vi "FPGA Main V3.vi"() -> ()   [LabVIEW 2018]
doc: "This VI reads all analogue data channels available at the fastest rate supported by the respective hardware and updates a memory address for when each measurement is available.\n\nAt a rate defined by the fastest module (NI 9237 - default of 12.5kHz) this memory is read, combined with the measurements from the 9237 module and written to the FIFO for communication to the RT machine.\n\nThe NI 9237 modeul therefore defines the nominal sampling rate of the system (with slower channels over-sampled).\n\nA time channel (in uSec) is provided with 0 referenced from the first acquisition of the NI 9237 module"
uses:
  <vilib>/LabVIEW Targets/FPGA/cRIO/shared/nicrio_ModuleControls/nicrio_cRIO-9237_DataRatesRing.ctl
  <vilib>/Platform/TimedLoop/XDataNode/timing_clust.ctl
  <vilib>/Platform/TimedLoop/XDataNode/nitl_modes.ctl
  <vilib>/Platform/TimedLoop/XDataNode/wakeup.ctl
  <vilib>/rvi/Emulation/niFpgaGetClockAttributes.vi
  <vilib>/rvi/Emulation/niFpgaSctlEmulationGetInTimedLoop.vi
  <vilib>/rvi/Emulation/niFpgaEmulationReportErrorSimple.vi
  <vilib>/rvi/Emulation/niFpgaProcessEmulError.vi
  <vilib>/rvi/eio/common/nirviEmuTemplatePropertySet_noerrors.vi
  <vilib>/rvi/eio/common/nirviEmuTemplateMethod_errors.vi
  <vilib>/rvi/interface/RandomDataEmulation/niFpgaRandomDataHandleErrors.vi
  <vilib>/rvi/Memory/Memory_Emulation/nirvimemoryFastEmulation.vi
  <vilib>/rvi/Memory/Memory_Emulation/nirvimemoryEmulation.vi
  <vilib>/rvi/Emulation/niFpgaEmulationIsFPGAContextNoSignature.vi
  <vilib>/rvi/DataTransferAndStorage/Container/Common/niFpgaContainerGetUniqueNameForEmu.vi
  <vilib>/rvi/errors/nirviReportUnexpectedCaseInternalError (U32).vi
  <vilib>/rvi/Emulation/niFpgaCriticalErrorInLSC.vi
  <vilib>/rvi/FIFO/Fifo_Resource/nirvififoEmulationSetSize.vi
  <vilib>/rvi/FIFO/Fifo_Resource/nirviFifoEmulationQueueMgr.vi
  <instcachedir>/0/nirviFifoEmulationQueueMgr_E5CAEC123FF24DC58D834DCA3CDAA9B5.lvgen/nirviFifoEmulationQueueMgr_E5CAEC123FF24DC58D834DCA3CDAA9B5_002.vi
  <vilib>/rvi/errors/niFpgaSetErrorForExecOnDevCompSimple.vi
  <vilib>/rvi/eio/common/nirviEmuReportErrorAndStop.vi
  <vilib>/Utility/error.llb/Clear Errors.vi
  <vilib>/rvi/FIFO/Fifo_Resource/nirvififoEmulationCreateLock.vi
  <vilib>/rvi/FIFO/Fifo_Resource/nirvififoEmulationObtainLock.vi
  <vilib>/rvi/FIFO/Fifo_Resource/nirvififoEmulationReleaseLock.vi
  <vilib>/rvi/occurrence/nirviWaitOnOccurrenceBase.vi
  <vilib>/rvi/errors/nirviReportUnexpectedCaseInternalError.vi
  <vilib>/rvi/FIFO/Fifo_Resource/nirvififoEmulationDetermineInputValidOut.vi
  <vilib>/eio/EIOPropertyNode/EIOPropertyNode.xnode
  <vilib>/eio/EIONode/EIONode.xnode
  <vilib>/rvi/DataTransferAndStorage/Container/XNode/niFpgaContainer.xnode
  <vilib>/rvi/interface/RandomDataEmulation/nirviRandomDataFpgaReadWriteTemplate.vi
  <vilib>/rvi/FIFO/Fifo_Resource/nirvififoEmulationGetNumberOfElementsToRead.vi
  <vilib>/rvi/FIFO/Fifo_Resource/nirvififoEmulationRead.vi
  <vilib>/eio/EIOMethodNode/EIOMethodNode.xnode
  <vilib>/platform/TimedLoop/XDataNode/XDataNode.xnode
  <vilib>/rvi/FIFO/Fifo_Resource/nirvififoEmulationWrite.vi
  <vilib>/Platform/TimedLoop/XDataNode/XDNodeRunTimeDep.lvlib
  <vilib>/rvi/eio/common/nirviEmuTemplatePropertyGet_errors.vi
  <vilib>/rvi/eio/common/nirviEmuTemplatePropertyGet_noerrors.vi
  <vilib>/rvi/eio/common/nirviEmuTemplatePropertySet_errors.vi
panel:
  in  "speedOutputScaling":sgl=6366198.0
  out "Speed":sgl caption="Speed (rads/tick)"
  out "filteredAngle":sgl caption="filteredAngle (rads)"
  out "filteredSpeed":sgl
  out "S1":u32
  in  "Edge filter":T1={"filterSize"=50, "lowerThreshold"=5, "upperThreshold"=45}
  out "edge separation":u32 caption="edge separation (ticks)"
  in  "falling edge (F)":bool caption="Torque encoder direction"
  in  "switch encoders":bool
  in  "Data Rate":T2=1 items=["50.000 kS/s (NI 9237)"=1, "25.000 kS/s (NI 9237)"=2, "16.667 kS/s (NI 9237)"=3, "12.500 kS/s (NI 9237)"=4, "10.000 kS/s (NI 9237)"=5, "8.333 kS/s (NI 9237)"=6, "7.143 kS/s (NI 9237)"=7, "6.250 kS/s (NI 9237)"=8, "5.556 kS/s (NI 9237)"=9, "5.000 kS/s (NI 9237)"=10, "4.545 kS/s (NI 9237)"=11, "4.167 kS/s (NI 9237)"=12, "3.846 kS/s (NI 9237)"=13, "3.571 kS/s (NI 9237)"=14, "3.333 kS/s (NI 9237)"=15, "3.125 kS/s (NI 9237)"=16, "2.941 kS/s (NI 9237)"=17, "2.778 kS/s (NI 9237)"=18, "2.632 kS/s (NI 9237)"=19, "2.500 kS/s (NI 9237)"=20, "2.381 kS/s (NI 9237)"=21, "2.273 kS/s (NI 9237)"=22, "2.174 kS/s (NI 9237)"=23, "2.083 kS/s (NI 9237)"=24, "2.000 kS/s (NI 9237)"=25, "1.923 kS/s (NI 9237)"=26, "1.852 kS/s (NI 9237)"=27, "1.786 kS/s (NI 9237)"=28, "1.724 kS/s (NI 9237)"=29, "1.667 kS/s (NI 9237)"=30, "1.613 kS/s (NI 9237)"=31]
  out "Total channel count":u32=61
  out "timestamp":u32
  out "FIFO full counter":i32
  in  "Safe Voltage":fxp<+/-,20,5>[](array[numeric])=[0.0, 0.0, 0.0, 0.0]
  in  "Safe Digital":bool[](array[boolean])=[FALSE, FALSE, FALSE, FALSE, FALSE, FALSE, FALSE, FALSE]
  in  "Voltage Out":fxp<+/-,20,5>[](array[numeric])=[0.0, 0.0, 0.0, 0.0]
  in  "Update Outputs":bool
  in  "Mod 8":bool[](array[boolean])=[FALSE, FALSE, FALSE, FALSE, FALSE, FALSE, FALSE, FALSE]
  out "E Stop":bool
  in  "Stop acquire":bool
  # "Torque Measurement"
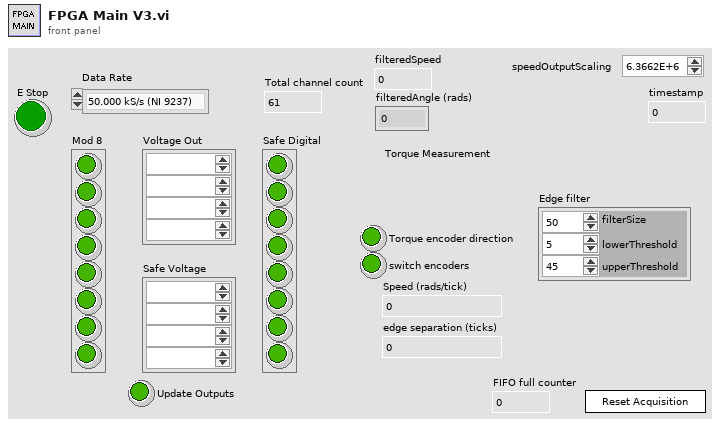
[diagram p1: front panel]
types:
  T1 = cluster{"filterSize":u8, "lowerThreshold":u8, "upperThreshold":u8}
  T2 = typedef "nicrio_cRIO-9237_DataRatesRing.ctl" = u8
  T3 = typedef "XDNodeRunTimeDep.lvlib/timing_clust.ctl" = cluster{"Expected End [f-1]":u64, "Actual End [f-1]":u64, "Finished Late? [f-1]":bool, "Expected End [i-1]":u64, "Actual End [i-1]":u64, "Finished Late? [i-1]":bool, "Expected Start [i]":u64, "Actual Start [i]":u64, "Expected Start [f]":u64, "Actual Start [f]":u64, "Source Name":string, "Structure Name":string, "Period":i64, "Deadline":i64, "Offset":i64, "Start":i64, "Priority":i32, "Timeout":i32, "Mode":T4, "Wakeup Reason":T5, "Error":errorcluster, "Source Type":string, "Secondary Source Type":string, "Global End Time":u64, "Global Start Time":u64, "Frame Duration":u64, "Iteration Duration":u64, "Assigned CPU":i32, "I/O Scan Engine Mode":u32}
  T4 = typedef "XDNodeRunTimeDep.lvlib/nitl_modes.ctl" = enum32{"No Change", "Process missed periods, maintain original phase", "Discard missed periods, maintain original phase", "Process missed periods, ignore original phase", "Discard missed periods, ignore original phase"}
  T5 = typedef "XDNodeRunTimeDep.lvlib/wakeup.ctl" = enum32{"Normal", "Aborted", "Asynchronous wakeup", "Timing source error", "Timed loop error", "Timeout"}
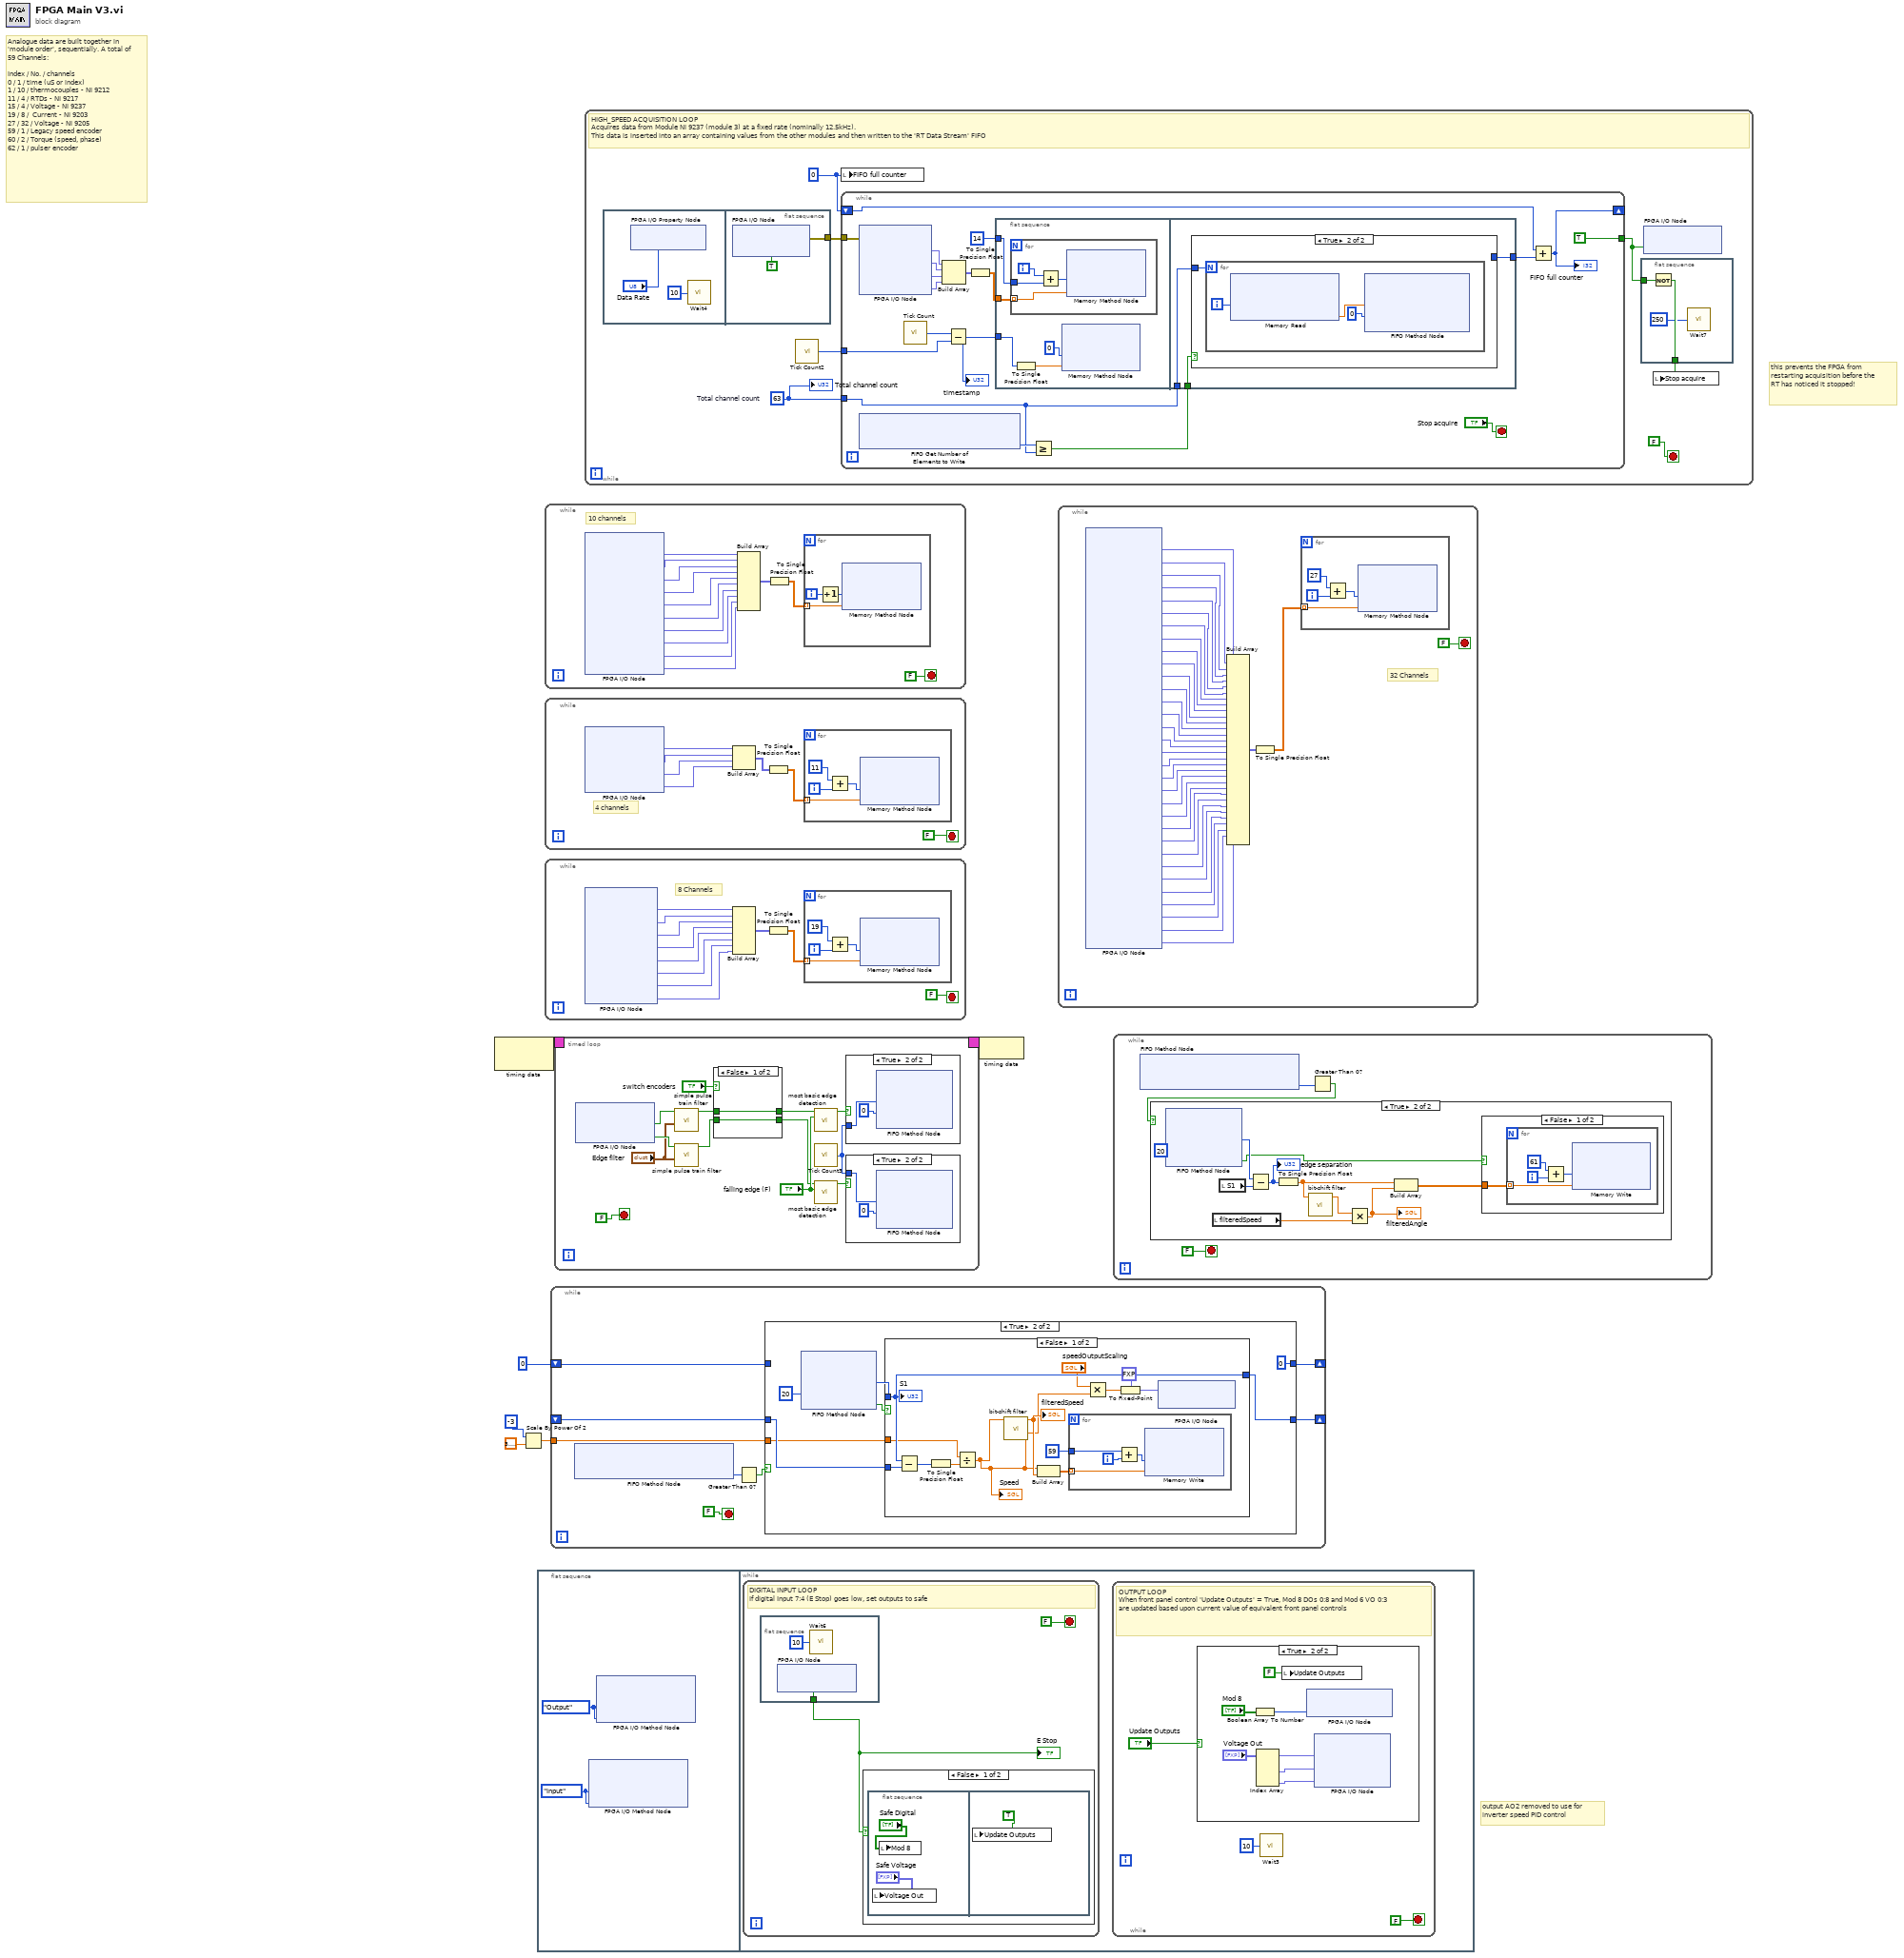
[diagram p0: block diagram]
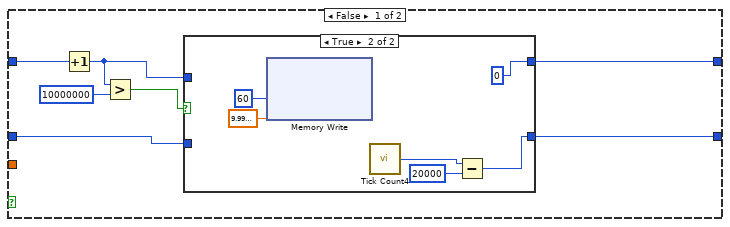
[diagram p4: hidden frame]
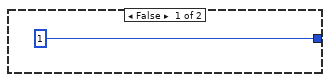
[diagram p12: hidden frame]
diagram:
  # "output AO2 removed to use for inverter speed PID control"
  # "this prevents the FPGA from restarting acquisition before the RT has noticed it stopped!"
  # "Analogue data are built together in 'module order', sequentially. A total of 59 Channels:\n\nIndex / No. / channels\n0 / 1 / time (uS or index)\n1 / 10 / thermocouples - NI 9212\n11 / 4 / RTDs - NI 9217\n15 / 4 / Voltage - NI 9237\n19 / 8 /  Current - NI 9203\n27 / 32 / Voltage - NI 9205\n59 / 1 / Legacy speed encoder\n60 / 2 / Torque (speed, phase)\n62 / 1 / pulser encoder"
  n1 = node-c288() -> (w6:T3)  [unwired: 1 in]
  n2 = Scale By Power Of 2(n=i16 -3, x=sgl 3.1415927) -> (x*2^n=w2:sgl)
  n3 = flat-sequence {
    frame #0 {
      w7 = enum8{"No Change", "Input", "Output"}."Output" ("DIO 7:4")
      w8 = enum8{"No Change", "Input", "Output"}."Input" ("DIO 7:4")
      n4 = xnode "FPGA I/O Method Node"("DIO 7:4"=w8, "DIO 3:0"=w8) -> ()  [unwired: 1 in, 1 out]
      n5 = xnode "FPGA I/O Method Node"("DIO 7:4"=w7, "DIO 3:0"=w7) -> ()  [unwired: 1 in, 1 out]
    }
    frame #1 {
      n6 = while {
        stop <- FALSE stop-if-true
        # "DIGITAL INPUT LOOP\nIf digital Input 7:4 (E Stop) goes low, set outputs to safe"
        n7 = flat-sequence {
          tunnel: [w22] -> w19
          frame #0 {
            n8 = xnode "FPGA I/O Node"() -> ("Mod7/DIO4"=w22:bool)  [unwired: 1 in, 1 out]
            n9 = call "Wait6"("Count(uSec)"=u8 10) -> ()  [unwired: 1 out]
          }
        }
        n10 = case shown="False" w19 {
          frame False {
            n11 = flat-sequence {
              frame #0 {
                n12 = local write "Voltage Out"("Safe Voltage") -> ()
                n13 = local write "Mod 8"("Safe Digital") -> ()
              }
              frame #1 {
                n14 = local write "Update Outputs"(TRUE ("Update Outputs")) -> ()
              }
            }
          }
          frame True {
          }
        }
        "E Stop" <- w19
      }
      n15 = while {
        stop <- FALSE stop-if-true
        # "OUTPUT LOOP\nWhen front panel control 'Update Outputs' = True, Mod 8 DOs 0:8 and Mod 6 VO 0:3 are updated based upon current value of equivalent front panel controls"
        n16 = case shown="True" "Update Outputs" {
          frame False {
          }
          frame True {
            n17 = Boolean Array To Number(Boolean array="Mod 8") -> (number=w17:u8)
            n18 = Index Array(array="Voltage Out") -> (element #1=w15:fxp<+/-,20,5>, element #2=w14:fxp<+/-,20,5>, element #4=w13:fxp<+/-,20,5>)  [unwired: 4 in, 1 out]
            n19 = local write "Update Outputs"(FALSE ("Update Outputs")) -> ()
            n20 = xnode "FPGA I/O Node"("Mod8/DIO7:0"=w17) -> ()  [unwired: 1 in, 1 out]
            n21 = xnode "FPGA I/O Node"("Mod6/AO0"=w15, "Mod6/AO1"=w14, "Mod6/AO3"=w13) -> ()  [unwired: 3 in, 3 out]
          }
        }
        n22 = call "Wait3"("Count(uSec)"=u16 10 ("Count(Ticks)")) -> ()  [unwired: 1 out]
      }
    }
  }
  n23 = while {
    stop <- FALSE stop-if-true
    # "10 channels"
    n24 = xnode "FPGA I/O Node"() -> ("Mod1/TC0"=w38:fxp<+/-,24,-2>, "Mod1/TC1"=w37:fxp<+/-,24,-2>, "Mod1/TC2"=w36:fxp<+/-,24,-2>, "Mod1/TC3"=w35:fxp<+/-,24,-2>, "Mod1/TC4"=w34:fxp<+/-,24,-2>, "Mod1/TC5"=w33:fxp<+/-,24,-2>, "Mod1/TC6"=w32:fxp<+/-,24,-2>, "Mod1/TC7"=w31:fxp<+/-,24,-2>, "Mod1/CJC0"=w28:fxp<+/-,24,-2>, "Mod1/CJC1"=w27:fxp<+/-,24,-2>)  [unwired: 10 in, 10 out]
    n25 = Build Array(w38, w37, w36, w35, w34, w33, w32, w31, w28, w27) -> (w30:fxp<+/-,24,-2>[])
    n26 = To Single Precision Float(number=w30) -> (single precision float=w29:sgl[])
    n27 = for {
      tunnel: w29 -> [w41] mode=indexing
      i -> [w40]
      n28 = Increment(x=w40) -> (x+1=w39:i32)
      n29 = xnode ("Memory Method Node")("Address"=w39, "Data"=w41) -> ()  [unwired: 1 in, 1 out]
    }
  }
  n30 = while {
    stop <- FALSE stop-if-true
    # "4 channels"
    n31 = xnode "FPGA I/O Node"() -> ("Mod2/RTD0"=w48:fxp<+/-,24,10>, "Mod2/RTD1"=w47:fxp<+/-,24,10>, "Mod2/RTD2"=w46:fxp<+/-,24,10>, "Mod2/RTD3"=w43:fxp<+/-,24,10>)  [unwired: 4 in, 4 out]
    n32 = Build Array(w48, w47, w46, w43) -> (w45:fxp<+/-,24,10>[])
    n33 = To Single Precision Float(number=w45) -> (single precision float=w44:sgl[])
    n34 = for {
      tunnel: w44 -> [w52] mode=indexing
      i -> [w51]
      n35 = Add(x=11 ("Numeric"), y=w51) -> (x+y=w50:i32)
      n36 = xnode ("Memory Method Node")("Address"=w50, "Data"=w52) -> ()  [unwired: 1 in, 1 out]
    }
  }
  n37 = while {
    stop <- FALSE stop-if-true
    # "8 Channels"
    n38 = xnode "FPGA I/O Node"() -> ("Mod4/AI0"=w63:fxp<+/-,21,-4>, "Mod4/AI1"=w62:fxp<+/-,21,-4>, "Mod4/AI2"=w61:fxp<+/-,21,-4>, "Mod4/AI3"=w58:fxp<+/-,21,-4>, "Mod4/AI4"=w57:fxp<+/-,21,-4>, "Mod4/AI5"=w56:fxp<+/-,21,-4>, "Mod4/AI6"=w55:fxp<+/-,21,-4>, "Mod4/AI7"=w54:fxp<+/-,21,-4>)  [unwired: 8 in, 8 out]
    n39 = Build Array(w63, w62, w61, w58, w57, w56, w55, w54) -> (w60:fxp<+/-,21,-4>[])
    n40 = To Single Precision Float(number=w60) -> (single precision float=w59:sgl[])
    n41 = for {
      tunnel: w59 -> [w67] mode=indexing
      i -> [w66]
      n42 = Add(x=19 ("Numeric"), y=w66) -> (x+y=w65:i32)
      n43 = xnode ("Memory Method Node")("Address"=w65, "Data"=w67) -> ()  [unwired: 1 in, 1 out]
    }
  }
  n44 = while {
    shift-right: [w74] -> _
    shift-left: _ -> [w73]
    tunnel: w2 -> [w72]
    shift-right: [w68] -> _
    shift-left: u32 0 ("n") -> [w69]
    stop <- FALSE stop-if-true
    n45 = xnode ("FIFO Method Node")() -> ("Number of Elements to Read"=w71:u32)  [unwired: 1 in, 1 out]
    n46 = Greater Than 0?(x=w71) -> (x > 0?=w70:bool)
    n47 = case shown="True" w70 {
      tunnel: [w76 w92] -> w74
      tunnel: w73 -> [w80 w97]
      tunnel: w72 -> [_ w96]
      tunnel: w69 -> [w82 _]
      tunnel: [w77 u32 0 ("n")] -> w68
      frame False {
        n48 = Increment(x=w82) -> (x+1=w78:u32)
        n49 = Greater?(x=w78, y=u32 10000000) -> (0:w79:bool)
        n50 = case shown="True" w79 {
          tunnel: w80 -> [w83 _]
          tunnel: w78 -> [w84 _]
          tunnel: [w84 u32 0 ("n")] -> w77
          tunnel: [w83 w86] -> w76
          frame False {
          }
          frame True {
            n51 = xnode ("Memory Write")("Address"=u32 60, "Data"=sgl 1e-09) -> ()  [unwired: 1 in, 1 out]
            n52 = call "Tick Count4"() -> ("Tick Count(Ticks)"=w89:u32)
            n53 = Subtract(x=w89, y=u32 20000) -> (x-y=w86:u32)
          }
        }
      }
      frame True {
        n54 = xnode ("FIFO Method Node")("Timeout"=20) -> ("Element"=w94:u32, "Timed Out?"=w93:bool)  [unwired: 1 in, 1 out]
        n55 = case shown="False" w93 {
          tunnel: w97 -> [w110 w115]
          tunnel: w96 -> [w107 _]
          tunnel: w94 -> [w108 _]
          tunnel: [w108 w115] -> w92
          frame False {
            n56 = Subtract(x=w108, y=w110) -> (x-y=w106:u32)
            n57 = To Single Precision Float(number=w106) -> (single precision float=w105:sgl)
            n58 = Divide(x=w107, y=w105) -> (x/y=w98:sgl)
            "Speed" <- w98
            n59 = call "bit-shift filter.vi"("newValue"=w98) -> ("filteredValue"=w103:sgl)  [unwired: 10 in]
            "filteredSpeed" <- w103
            n60 = Build Array(w98, w103) -> (w104:sgl[])
            n61 = for {
              tunnel: u32 59 ("Address") -> [w114]
              tunnel: w104 -> [w113] mode=indexing
              i -> [w111]
              n62 = Add(x=w114, y=w111) -> (x+y=w112:u32)
              n63 = xnode ("Memory Write")("Address"=w112, "Data"=w113) -> ()  [unwired: 1 in, 1 out]
            }
            n64 = Multiply(x="speedOutputScaling", y=w98) -> (x*y=w101:sgl)
            n65 = To Fixed-Point(fixed-point type=fxp<+/-,20,5> 0.0 ("Mod6/AO2"), number=w101) -> (fixed-point=w100:fxp<+/-,20,5>)
            n66 = xnode "FPGA I/O Node"("Mod6/AO2"=w100) -> ()  [unwired: 1 in, 1 out]
            "S1" <- w108
          }
          frame True {
          }
        }
      }
    }
  }
  n67 = timed-loop {
    timing: w6 -> [_]
    timing-out: [_] -> w5
    stop <- FALSE stop-if-true
    n68 = xnode "FPGA I/O Node"() -> ("Mod7/DIO0"=w128:bool, "Mod7/DIO1"=w127:bool)  [unwired: 2 in, 2 out]
    n69 = call "simple pulse train filter.vi"("filter params"="Edge filter", "realState"=w128) -> ("filteredState"=w120:bool)  [unwired: 9 in]
    n70 = call "simple pulse train filter.vi"("filter params"="Edge filter", "realState"=w127) -> ("filteredState"=w122:bool)  [unwired: 9 in]
    n71 = case shown="False" "switch encoders" {
      tunnel: [w134 w135] -> w123
      tunnel: w122 -> [w134 w136]
      tunnel: [w133 w136] -> w121
      tunnel: w120 -> [w133 w135]
      frame False {
      }
      frame True {
      }
    }
    n72 = call "most basic edge detection.vi"("falling edge"="falling edge (F)", "pulse"=w121) -> ("edge detected"=w119:bool)  [unwired: 9 in]
    n73 = call "Tick Count3"() -> ("Tick Count(Ticks)"=w116:u32)
    n74 = call "most basic edge detection.vi"("falling edge"="falling edge (F)", "pulse"=w123) -> ("edge detected"=w117:bool)  [unwired: 9 in]
    n75 = case shown="True" w119 {
      tunnel: w116 -> [_ w132]
      frame False {
      }
      frame True {
        n76 = xnode ("FIFO Method Node")("Element"=w132, "Timeout"=0) -> ()  [unwired: 1 in, 2 out]
      }
    }
    n77 = case shown="True" w117 {
      tunnel: w116 -> [_ w130]
      frame False {
      }
      frame True {
        n78 = xnode ("FIFO Method Node")("Element"=w130, "Timeout"=0) -> ()  [unwired: 1 in, 2 out]
      }
    }
  }
  n79 = while {
    stop <- FALSE stop-if-true
    w140 = 0 ("FIFO full counter")
    w143 = u32 63  # Total channel count
    # "HIGH_SPEED ACQUISITION LOOP\nAcquires data from Module NI 9237 (module 3) at a fixed rate (nominally 12.5kHz).\nThis data is inserted into an array containing values from the other modules and then written to the 'RT Data Stream' FIFO"
    n80 = flat-sequence {
      tunnel: [w152] -> w144
      frame #0 {
        n81 = xnode "FPGA I/O Property Node"("Data Rate"="Data Rate") -> ()  [unwired: 1 in, 1 out]
        n82 = call "Wait4"("Count(mSec)"=u16 10) -> ()  [unwired: 1 out]
      }
      frame #1 {
        n83 = xnode "FPGA I/O Node"("Mod3/Start"=TRUE) -> ("error out"=w152:errorcluster)  [unwired: 2 in, 1 out]
      }
    }
    n84 = call "Tick Count2"() -> ("Tick Count(uSec)"=w145:u32)
    n85 = local write "FIFO full counter"(w140) -> ()
    n86 = while {
      tunnel: [TRUE ("I/O Item")] -> w142
      tunnel: w144 -> [w170]
      tunnel: w143 -> [w155]
      shift-right: [w163] -> _
      shift-left: w140 -> [w161]
      tunnel: w145 -> [w164]
      stop <- "Stop acquire" stop-if-true
      n87 = xnode "FPGA I/O Node"("error in"=w170) -> ("Mod3/AI0"=w169:fxp<+/-,24,-4>, "Mod3/AI1"=w168:fxp<+/-,24,-4>, "Mod3/AI2"=w167:fxp<+/-,24,-4>, "Mod3/AI3"=w166:fxp<+/-,24,-4>)  [unwired: 4 in, 5 out]
      n88 = xnode ("FIFO Get Number of Elements to Write")() -> ("Number of Elements to Write"=w157:u32)  [unwired: 1 in, 1 out]
      n89 = call "Tick Count"() -> ("Tick Count(uSec)"=w160:u32)
      n90 = Build Array(w169, w168, w167, w166) -> (w165:fxp<+/-,24,-4>[])
      n91 = Subtract(x=w160, y=w164) -> (x-y=w153:u32)
      "timestamp" <- w153
      n92 = To Single Precision Float(number=w165) -> (single precision float=w159:sgl[])
      n93 = flat-sequence {
        tunnel: w159 -> [w176]
        tunnel: 14 ("index") -> [w175]
        tunnel: w153 -> [w173]
        tunnel: w155 -> [w183]
        tunnel: [w182] -> w154
        tunnel: w156 -> [w181]
        frame #0 {
          n94 = for {
            tunnel: w176 -> [w180] mode=indexing
            tunnel: w175 -> [w179]
            i -> [w177]
            n95 = Add(x=w177, y=w179) -> (x+y=w178:i32)
            n96 = xnode ("Memory Method Node")("Address"=w178, "Data"=w180) -> ()  [unwired: 1 in, 1 out]
          }
          n97 = To Single Precision Float(number=w173) -> (single precision float=w174:sgl)
          n98 = xnode ("Memory Method Node")("Address"=u32 0, "Data"=w174) -> ()  [unwired: 1 in, 1 out]
        }
        frame #1 {
          n99 = case shown="True" w181 {
            tunnel: [1 _] -> w182
            tunnel: w183 -> [_ w185]
            frame False {
            }
            frame True {
              n100 = for {
                N: w185 -> [_]
                i -> [w186]
                n101 = xnode ("Memory Read")("Address"=w186) -> ("Data"=w187:sgl)  [unwired: 1 in, 1 out]
                n102 = xnode ("FIFO Method Node")("Element"=w187, "Timeout"=0) -> ()  [unwired: 1 in, 2 out]
              }
            }
          }
        }
      }
      n103 = Greater Or Equal?(x=w157, y=w155) -> (x >= y?=w156:bool)
      n104 = Add(x=w161, y=w154) -> (x+y=w163:i32)
      "FIFO full counter" <- w163
    }
    n105 = flat-sequence {
      tunnel: w142 -> [w148]
      tunnel: [w147] -> w139
      frame #0 {
        n106 = Not(x=w148) -> (.not. x?=w147:bool)
        n107 = call "Wait7"("Count(mSec)"=u8 250) -> ()  [unwired: 1 out]
      }
    }
    n108 = xnode "FPGA I/O Node"("Mod3/Stop"=w142) -> ()  [unwired: 1 in, 1 out]
    n109 = local write "Stop acquire"(w139) -> ()
    "Total channel count" <- w143
  }
  n110 = node-c288(w5) -> ()
  n111 = while {
    stop <- FALSE stop-if-true
    # "32 Channels"
    n112 = xnode "FPGA I/O Node"() -> ("Mod5/AI0"=w191:fxp<+/-,26,5>, "Mod5/AI1"=w192:fxp<+/-,26,5>, "Mod5/AI2"=w193:fxp<+/-,26,5>, "Mod5/AI3"=w194:fxp<+/-,26,5>, "Mod5/AI4"=w195:fxp<+/-,26,5>, "Mod5/AI5"=w196:fxp<+/-,26,5>, "Mod5/AI6"=w197:fxp<+/-,26,5>, "Mod5/AI7"=w198:fxp<+/-,26,5>, "Mod5/AI8"=w222:fxp<+/-,26,5>, "Mod5/AI9"=w221:fxp<+/-,26,5>, "Mod5/AI10"=w220:fxp<+/-,26,5>, "Mod5/AI11"=w219:fxp<+/-,26,5>, "Mod5/AI12"=w218:fxp<+/-,26,5>, "Mod5/AI13"=w217:fxp<+/-,26,5>, "Mod5/AI14"=w216:fxp<+/-,26,5>, "Mod5/AI15"=w215:fxp<+/-,26,5>, "Mod5/AI16"=w214:fxp<+/-,26,5>, "Mod5/AI17"=w213:fxp<+/-,26,5>, "Mod5/AI18"=w212:fxp<+/-,26,5>, "Mod5/AI19"=w211:fxp<+/-,26,5>, "Mod5/AI20"=w210:fxp<+/-,26,5>, "Mod5/AI21"=w209:fxp<+/-,26,5>, "Mod5/AI22"=w208:fxp<+/-,26,5>, "Mod5/AI23"=w207:fxp<+/-,26,5>, "Mod5/AI24"=w206:fxp<+/-,26,5>, "Mod5/AI25"=w205:fxp<+/-,26,5>, "Mod5/AI26"=w204:fxp<+/-,26,5>, "Mod5/AI27"=w203:fxp<+/-,26,5>, "Mod5/AI28"=w202:fxp<+/-,26,5>, "Mod5/AI29"=w201:fxp<+/-,26,5>, "Mod5/AI30"=w200:fxp<+/-,26,5>, "Mod5/AI31"=w199:fxp<+/-,26,5>)  [unwired: 32 in, 32 out]
    n113 = Build Array(w191, w192, w193, w194, w195, w196, w197, w198, w222, w221, w220, w219, w218, w217, w216, w215, w214, w213, w212, w211, w210, w209, w208, w207, w206, w205, w204, w203, w202, w201, w200, w199) -> (w223:fxp<+/-,26,5>[])
    n114 = To Single Precision Float(number=w223) -> (single precision float=w190:sgl[])
    n115 = for {
      tunnel: w190 -> [w227] mode=indexing
      i -> [w226]
      n116 = Add(x=27 ("Numeric"), y=w226) -> (x+y=w225:i32)
      n117 = xnode ("Memory Method Node")("Address"=w225, "Data"=w227) -> ()  [unwired: 1 in, 1 out]
    }
  }
  n118 = while {
    stop <- FALSE stop-if-true
    n119 = xnode ("FIFO Method Node")() -> ("Number of Elements to Read"=w229:u32)  [unwired: 1 in, 1 out]
    n120 = Greater Than 0?(x=w229) -> (x > 0?=w228:bool)
    n121 = case shown="True" w228 {
      frame False {
      }
      frame True {
        n122 = xnode ("FIFO Method Node")("Timeout"=20) -> ("Element"=w237:u32, "Timed Out?"=w235:bool)  [unwired: 1 in, 1 out]
        n123 = local read "filteredSpeed"() -> (w234:sgl)
        n124 = local read "S1"() -> (w240:u32)
        n125 = Subtract(x=w237, y=w240) -> (x-y=w239:u32)
        "edge separation" <- w239
        n126 = To Single Precision Float(number=w239) -> (single precision float=w233:sgl)
        n127 = call "bit-shift filter.vi"("newValue"=w233) -> ("filteredValue"=w232:sgl)  [unwired: 10 in]
        n128 = Multiply(x=w232, y=w234) -> (x*y=w231:sgl)
        "filteredAngle" <- w231
        n129 = Build Array(w233, w231) -> (w238:sgl[])
        n130 = case shown="False" w235 {
          tunnel: w238 -> [w241 _]
          frame False {
            n131 = for {
              tunnel: w241 -> [w242] mode=indexing
              i -> [w244]
              n132 = Add(x=u32 61 ("Address"), y=w244) -> (x+y=w243:u32)
              n133 = xnode ("Memory Write")("Address"=w243, "Data"=w242) -> ()  [unwired: 1 in, 1 out]
            }
          }
          frame True {
          }
        }
      }
    }
  }
